vi "licht_op_groen (SubVI).vi"(8 "manuel override?":bool, 10 "Boolean":bool, 11 "OK Button":bool) -> (0 "manuel override":bool, 3 "licht op groen":bool)   [LabVIEW 2019]
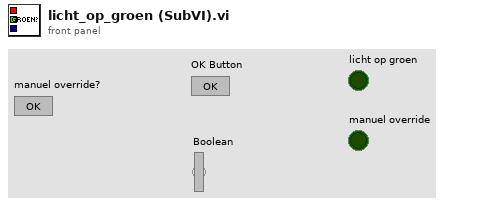
[diagram p1: front panel]
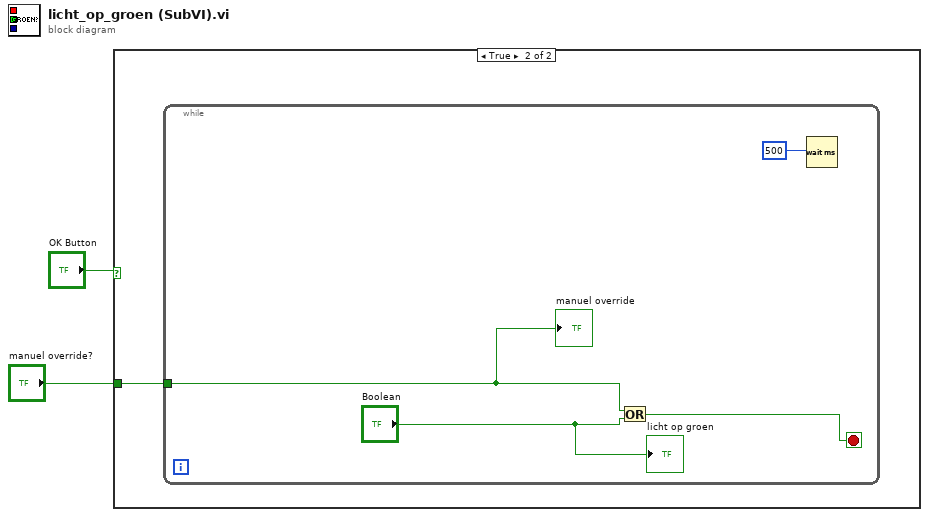
[diagram p0: block diagram]
diagram:
  n1 = case shown="True" "OK Button" {
    tunnel: "manuel override?" -> [_ w3]
    frame False {
    }
    frame True {
      n2 = while {
        tunnel: w3 -> [w4]
        stop <- w6 stop-if-true
        n3 = Or(x=w4, y="Boolean") -> (x .or. y?=w6:bool)
        n4 = Wait (ms)(milliseconds to wait=500) -> ()  [unwired: 1 out]
        "licht op groen" <- "Boolean"
        "manuel override" <- w4
      }
    }
  }
